vi "Start Executor.vi"(8 "error in (no error)":errorcluster, 11 "Future in":refnum<class "Future.lvclass">) -> (0 "error out":errorcluster, 3 "Future out":refnum<class "Future.lvclass">)   [LabVIEW 2017, in "Promise Future.lvlib" / "Future.lvclass"]
uses:
  Future.lvclass
  Callback/Callback.lvclass
  Future.lvclass/Future.ctl
  Callback/Blocking Callback.lvclass
  E:/Promise/Promise Future/Callback/Callback.lvclass
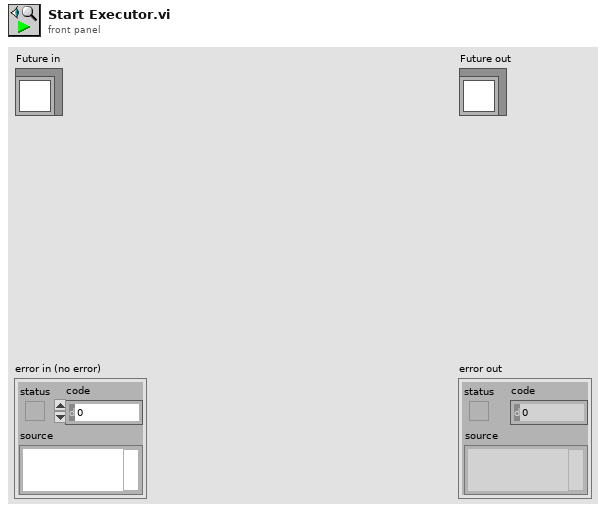
[diagram p1: front panel]
types:
  T1 = typedef "Semaphore RefNum" = refnum<k1>
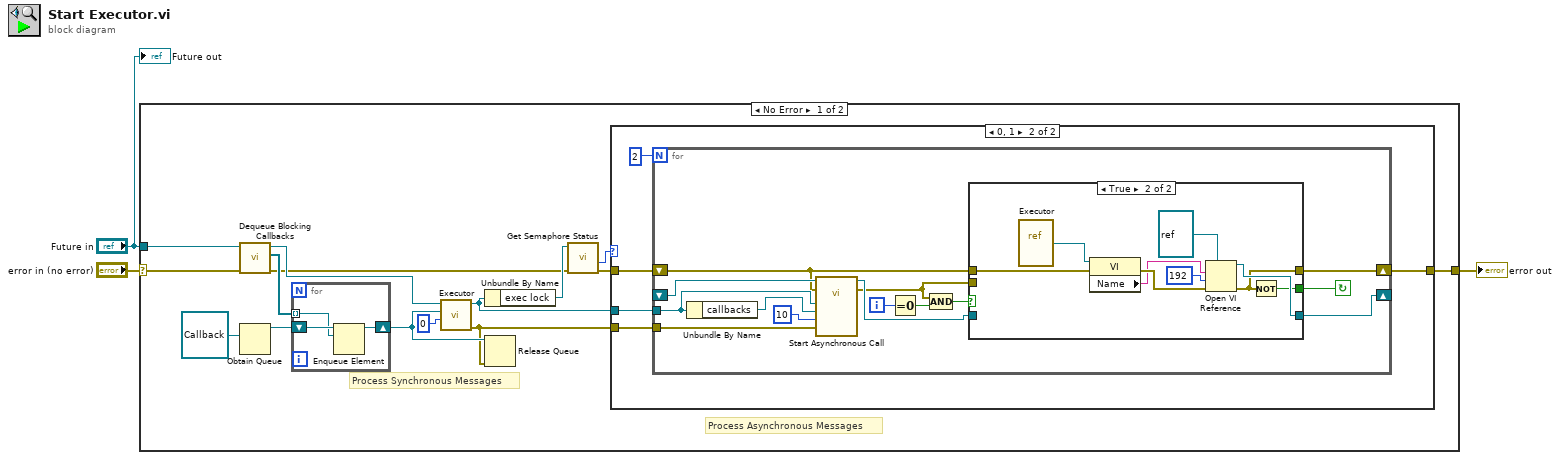
[diagram p0: block diagram]
diagram:
  n1 = case shown="No Error" "error in (no error)" {
    selector: "error in (no error)" -> [w14 w54]
    tunnel: [w18 w54] -> w2
    tunnel: "Future in" -> [w5 _]
    frame No Error {
      # "Process Asynchronous Messages"
      # "Process Synchronous Messages"
      n2 = call "Dequeue Blocking Callbacks.vi"("error in (no error)"=w14, "Future in"=w5) -> ("error out"=w7:errorcluster, "Sync Callbacks"=w11:refnum<class "Blocking Callback.lvclass">[], "Future out"=w13:refnum<class "Future.lvclass">)  [unwired: 7 in]
      n3 = Obtain Queue(element data type=refnum<class "Callback.lvclass"> refnum ("Promise Future.lvlib:Callback.lvclass")) -> (queue out=w10:refnum<queue>)  [unwired: 4 in, 2 out]
      n4 = for {
        tunnel: w11 -> [w19] mode=indexing
        shift-right: [w20] -> w8
        shift-left: w10 -> [w21]
        n5 = Enqueue Element(queue=w21, element=w19) -> (queue out=w20:refnum<queue>)  [unwired: 2 in, 2 out]
      }
      n6 = call "Executor.vi"("stay active on empty queue (ms)"=0 ("wait on queue in ms (-1)"), "callbacks"=w8, "Future"=w13) -> ("error out"=w6:errorcluster, "Future out"=w12:refnum<class "Future.lvclass">)  [unwired: 7 in]
      n7 = Unbundle By Name(w12) -> ("exec lock"=w17:T1)
      n8 = Release Queue(queue=w8, error in (no error)=w6) -> ()  [unwired: 1 in, 3 out]
      n9 = call <vilib>:"Get Semaphore Status.vi"("error in (no error)"=w7, "semaphore"=w17) -> ("error out"=w15:errorcluster, "# waiting"=w16:i32)  [unwired: 4 in, 4 out]
      n10 = case shown="0, 1" w16 {
        tunnel: [w22 w27] -> w18
        tunnel: w12 -> [_ w24]
        tunnel: w15 -> [w22 w26]
        tunnel: w6 -> [_ w23]
        frame Default {
          # "Already have another executor waiting for the queue, don't bother launching more"
        }
        frame 0, 1 {
          n11 = for {
            N: 2 -> [_]
            shift-right: [w41] -> _
            shift-left: _ -> [w33]
            shift-right: [w40] -> w27
            shift-left: w26 -> [w30]
            tunnel: w24 -> [w32]
            tunnel: w23 -> [w29]
            i -> [w37]
            stop <- w36 continue-if-true
            n12 = Unbundle By Name(w32) -> ("callbacks"=w31:refnum<queue>)
            n13 = call-by-ref "Start Asynchronous Call"(reference=w33, error in=w30, 8:"error in (no error)"=w29, "stay active on empty queue (ms)"=10 ("wait on queue in ms (-1)"), "callbacks"=w31, "Future"=w32) -> (reference out=w35:refnum<vi>, error out=w34:errorcluster)  [unwired: 6 in, 2 out]
            n14 = Equal To 0?(x=w37) -> (x = 0?=w38:bool)
            n15 = Compound Arithmetic op=AND(w34, w38) -> (w39:bool)
            n16 = case shown="True" w39 {
              selector: w39 -> [w42 _]
              tunnel: [w44 w50] -> w41
              tunnel: [w43 w48] -> w40
              tunnel: w35 -> [w44 _]
              tunnel: w34 -> [w43 _]
              tunnel: [w42 w49] -> w36
              tunnel: w30 -> [_ w47]
              frame False {
              }
              frame True {
                n17 = vi-ref "Executor.vi"() -> (w46:refnum<vi>)
                n18 = property class="VI"(reference=w46, error in=w47) -> (error out=w53:errorcluster, "Name"=w52:string)  [unwired: 1 out]
                n19 = Open VI Reference(type specifier VI Refnum (for type only)=refnum<vi> refnum, vi path=w52, options=192, error in (no error)=w53) -> (vi reference=w50:refnum<vi>, error out=w48:errorcluster)  [unwired: 2 in]
                n20 = Not(x=w48) -> (.not. x?=w49:bool)
              }
            }
          }
        }
      }
    }
    frame Error {
    }
  }
  "error out" <- w2
  "Future out" <- "Future in"
